vi "helper-eng-rec.vi"(11 "input cluster":T1 {"IOnode"."calibration"."Y" format="%#.3f"; "IOnode"."calibration"."X" format="%#.3f"; "IOnode"."ADDR" format="%04d"}) -> (0 "error":errorcluster)   [LabVIEW 2024]
uses:
  controls/cluster-com-log.ctl
  controls/IONode.ctl
  controls/type.address.ctl
  controls/enum.io.type.ctl
  controls/enum.io.mode.ctl
  controls/typeXyPoint.ctl
  <vilib>/Utility/error.llb/Trim Whitespace.vi
  <vilib>/Utility/error.llb/Trim Whitespace One-Sided.vi
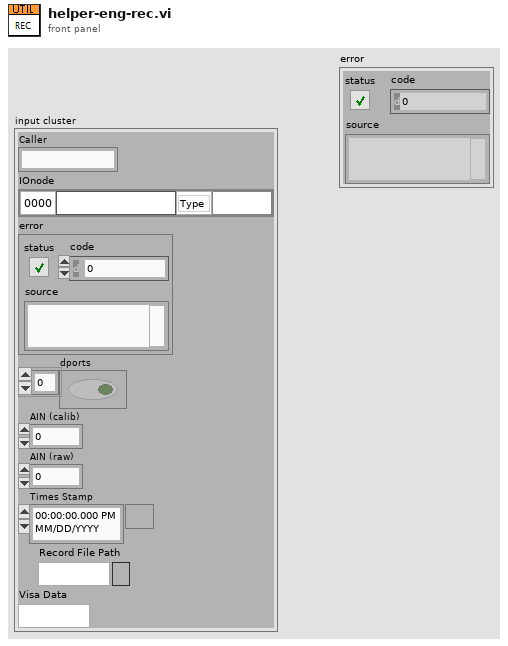
[diagram p1: front panel]
types:
  T1 = typedef "cluster-com-log.ctl" = cluster{"Caller":string, "IOnode":T2, "error":errorcluster, "dports":bool[], "AIN (calib)":dbl, "AIN (raw)":u16, "Times Stamp":timestamp, "Record File Path":path, "Visa Data":string}
  T2 = typedef "IONode.ctl" = cluster{"ADDR":T3, "Label":string, "Type":T4, "Mode":T5, "Value":string, "Tags":string, "calibration":T6[]}
  T3 = typedef "type.address.ctl" = u16
  T4 = typedef "enum.io.type.ctl" = enum16{"Type", "DI", "DO", "AI", "AO", "VL", "BUF"}
  T5 = typedef "enum.io.mode.ctl" = enum16{"Mode", "RIO", "SIM"}
  T6 = typedef "typeXyPoint.ctl" = cluster{"X":dbl, "Y":dbl}
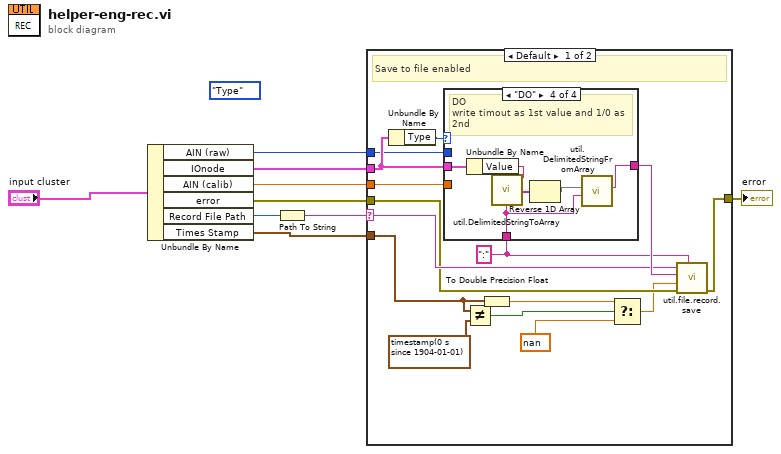
[diagram p0: block diagram]
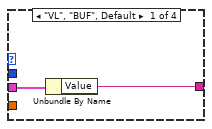
[diagram p2: hidden frame]
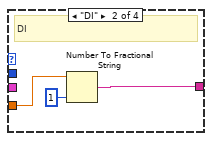
[diagram p3: hidden frame]
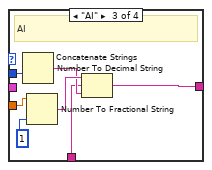
[diagram p4: hidden frame]
diagram:
  (unwired) enum.io.type."Type" ("Type")
  n1 = Unbundle By Name("input cluster") -> ("AIN (raw)"=w8:u16, "IOnode"=w7:T2, "AIN (calib)"=w9:dbl, "error"=w1:errorcluster, "Record File Path"=w5:path, "Times Stamp"=w3:timestamp)
  n2 = Path To String(path=w5) -> (string=w4:string)
  n3 = case shown="Default" w4 {
    selector: w4 -> [w18 _]
    tunnel: [w22 _] -> w2
    tunnel: w9 -> [w24 _]
    tunnel: w7 -> [w23 _]
    tunnel: w8 -> [w21 _]
    tunnel: w3 -> [w10 _]
    tunnel: w1 -> [w16 _]
    frame Default {
      w17 = ":" ("string")
      # "Save to file enabled"
      n4 = Unbundle By Name(w23) -> ("Type"=w20:T4)
      n5 = case shown="\"DO\"" w20 {
        tunnel: w24 -> [_ w28 w35 _]
        tunnel: w23 -> [w26 _ _ w42]
        tunnel: [w25 w27 w32 w37] -> w19
        tunnel: w21 -> [_ _ w34 _]
        tunnel: w17 -> [_ _ w30 w40]
        frame "VL", "BUF", Default {
          n6 = Unbundle By Name(w26) -> ("Value"=w25:string)
        }
        frame "DI" {
          # "DI"
          n7 = Number To Fractional String(number=w28, precision (6)=i16 1) -> (F-format string=w27:string)  [unwired: 2 in]
        }
        frame "AI" {
          # "AI"
          n8 = Number To Decimal String(number=w34) -> (decimal integer string=w31:string)  [unwired: 1 in]
          n9 = Number To Fractional String(number=w35, precision (6)=i16 1) -> (F-format string=w33:string)  [unwired: 2 in]
          n10 = Concatenate Strings(w33, w30, w31) -> (w32:string)
        }
        frame "DO" {
          # "DO\nwrite timout as 1st value and 1/0 as 2nd"
          n11 = Unbundle By Name(w42) -> ("Value"=w38:string)
          n12 = call "util.DelimitedStringToArray.vi"("delimiter (,)"=w40, "delimitaed string"=w38) -> ("array out"=w41:string[])  [unwired: 9 in]
          n13 = Reverse 1D Array(array=w41) -> (reversed array=w39:string[])
          n14 = call "util.DelimitedStringFromArray.vi"("delimiter (Comma)"=w40, "params array in"=w39) -> ("delimited string out"=w37:string)  [unwired: 9 in]
        }
      }
      n15 = Not Equal?(x=w10, y=timestamp(0 s since 1904-01-01)) -> (x != y?=w15:bool)
      n16 = To Double Precision Float(number=w10) -> (double precision float=w12:dbl)
      n17 = Select(t=w12, s=w15, f=nan) -> (s? t:f=w11:dbl)
      n18 = call "util.file.record.save.vi"("delimiter (,)"=w17, "error in"=w16, "clk(NaN)"=w11, "String Delimited Values"=w19, "record path in"=w18) -> ("error out"=w22:errorcluster)  [unwired: 5 in, 1 out]
    }
    frame "" {
      # "Save to file disabled"
    }
  }
  "error" <- w2
